vi "Forces Get.vi"(8 "error in (no error)":errorcluster) -> (0 "error out":errorcluster, 2 "Force (N)":T1 {"Fz (N)" format="%.1f"; "Fy (N)" format="%.1f"; "Fx (N)" format="%.1f"})   [LabVIEW 2022 SP3, in "Haptic Prog Interface.lvlib"]
doc: "Returns the forces of the haptic pen in N.\n\n<b>Force:</b> Returns a cluster of the x, y, and z forces on the pen (in units of N)."
uses:
  Haptic Prog Interface.lvlib
  Haptic-Programming-Interface/src/x64/Debug/Haptic Programming Interface.dll
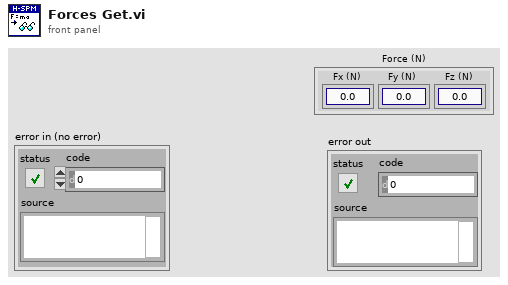
[diagram p1: front panel]
types:
  T1 = cluster{"Fx (N)":dbl, "Fy (N)":dbl, "Fz (N)":dbl}
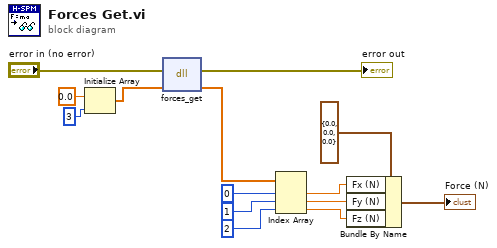
[diagram p0: block diagram]
diagram:
  n1 = Initialize Array(0.0 ("element"), 3 ("dimension size")) -> (w1:dbl[])
  n2 = dll-call lib="C:/Users/cjwel/Documents/GitHub/Haptic-Programming-Interface/src/x64/Debug/Haptic Programming Interface.dll" fn="forces_get"(error in="error in (no error)", "output"=w1) -> (error out=→"error out":errorcluster, "output"=w12:dbl[])  [unwired: 3 in, 1 out]
  n3 = Index Array(array=w12, index #1=0 ("index"), index #2=1 ("index"), index #3=2 ("index")) -> (element #1=w6:dbl, element #2=w8:dbl, element #3=w7:dbl)
  n4 = Bundle By Name(cluster=T1 {"Fx (N)"=0.0, "Fy (N)"=0.0, "Fz (N)"=0.0} ("Forces"), "Fx (N)"=w6, "Fy (N)"=w8, "Fz (N)"=w7) -> (→"Force (N)":T1)
